vi "LeerBaseDatos_interno.vi"(8 "error in (no error)":errorcluster, 11 "Prueba01 in":refnum<class "Prueba01.lvclass">) -> (0 "error out":errorcluster, 3 "Prueba01 out":refnum<class "Prueba01.lvclass">)   [LabVIEW 2019, in "Prueba01.lvclass"]
uses:
  Prueba01.lvclass
  Controles/BD_P01.ctl
  Prueba01.lvclass/Prueba01.ctl
  Base de Datos/SQLiteConnector/SQLiteConnection.lvclass
  Base de Datos/Base de Datos.lvclass
panel:
  out "BD":T1
  in  "Tipo Equipo":enum16{"Sonometro", "Calibrador", "Dosimetro"}(ring)
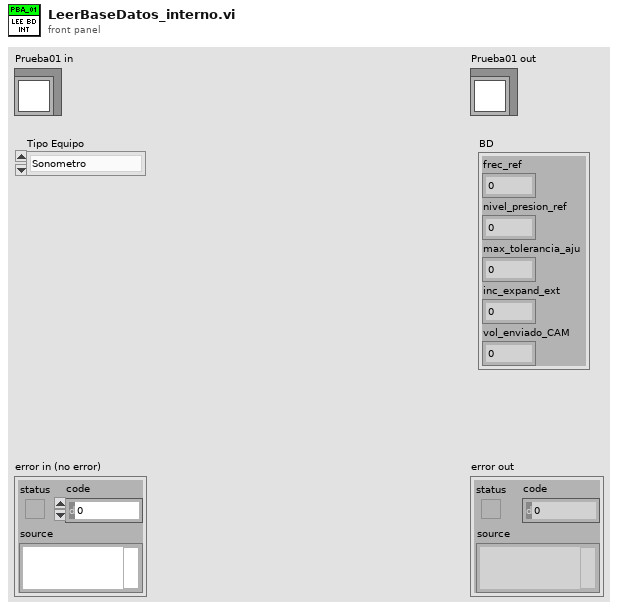
[diagram p1: front panel]
types:
  T1 = typedef "Prueba01.lvclass/BD_P01.ctl" = cluster{"frec_ref":dbl, "nivel_presion_ref":dbl, "max_tolerancia_aju":dbl, "inc_expand_ext":dbl, "vol_enviado_CAM":dbl}
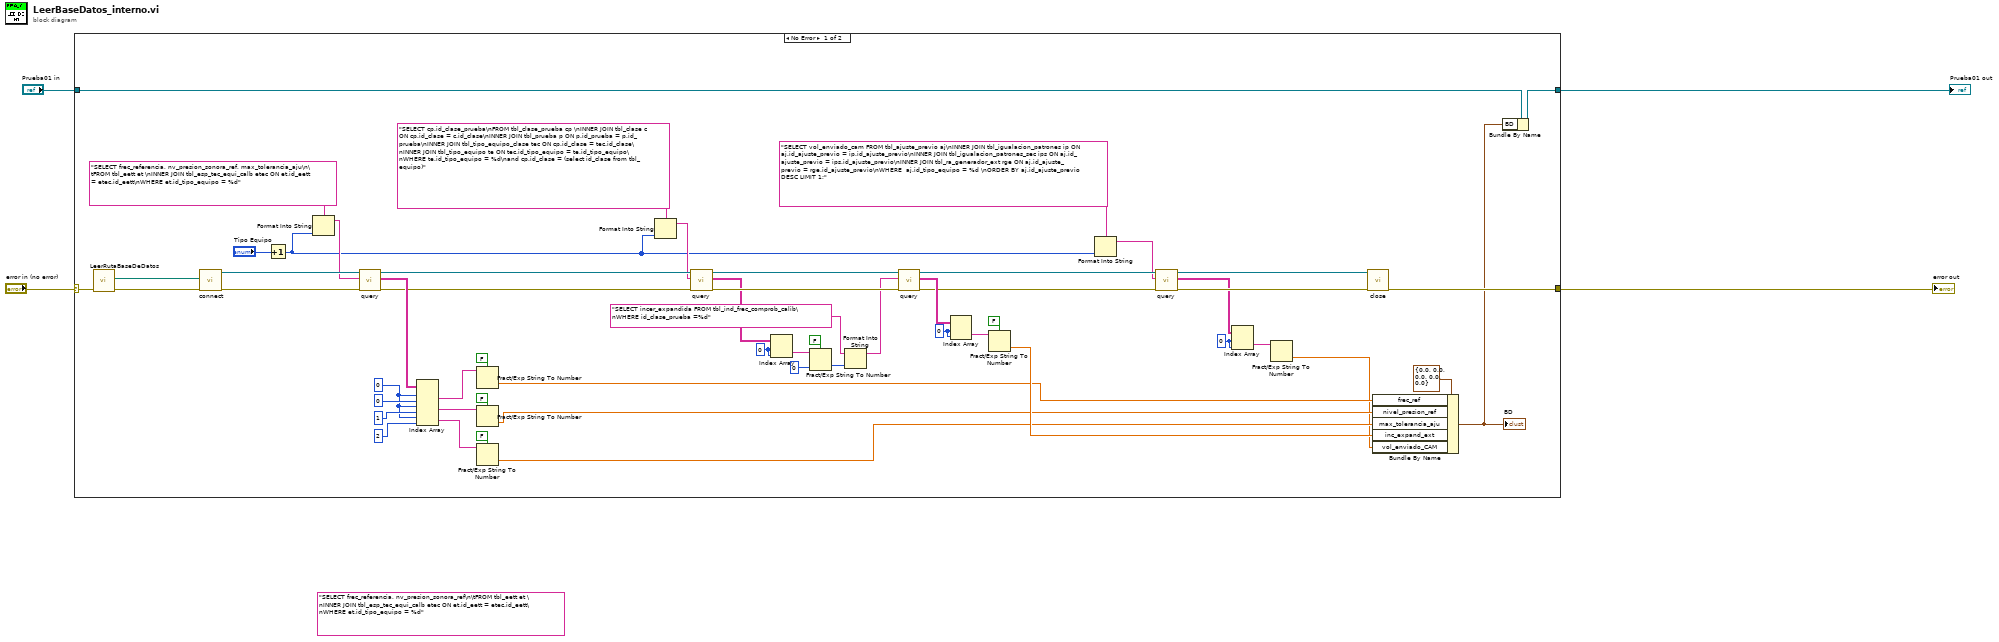
[diagram p0: block diagram]
diagram:
  (unwired) "SELECT frec_referencia, nv_presion_sonora_ref\n\tFROM tbl_eett et \nINNER JOIN tbl_esp_tec_equi_calb etec ON et.id_eett = etec.id_eett\nWHERE et.id_tipo_equipo = %d" ("format string")
  n1 = case shown="No Error" "error in (no error)" {
    selector: "error in (no error)" -> [w60 w63]
    tunnel: [w52 w63] -> w3
    tunnel: [w17 w62] -> w1
    tunnel: "Prueba01 in" -> [w61 w62]
    frame No Error {
      w8 = 0 ("index (row)")
      w24 = 0 ("index (row)")
      w35 = 0 ("index (row)")
      w44 = 0 ("index (row)")
      n2 = call "LeerRutaBaseDeDatos.vi"("error in (no error)"=w60) -> ("error out"=w54:errorcluster, "Database Path"=w53:path)  [unwired: 9 in]
      n3 = call "connect.vi"("error in (no error)"=w54, "Database Path"=w53) -> ("error out"=w56:errorcluster, "object out"=w57:refnum<class "SQLiteConnection.lvclass">)  [unwired: 8 in]
      n4 = Increment(x="Tipo Equipo") -> (x+1=w9:enum16{"Sonometro", "Calibrador", "Dosimetro"})
      n5 = Format Into String(format string="SELECT frec_referencia, nv_presion_sonora_ref, max_tolerancia_aju\n\tFROM tbl_eett et \nINNER JOIN tbl_esp_tec_equi_calb etec ON et.id_eett = etec.id_eett\nWHERE et.id_tipo_equipo = %d", w9) -> (resulting string=w55:string)  [unwired: 2 in, 1 out]
      n6 = call "query.vi"("error in (no error)"=w56, "SQL Statement"=w55, "object in"=w57) -> ("error out"=w40:errorcluster, "result"=w51:string[][], "object out"=w39:refnum<class "SQLiteConnection.lvclass">)  [unwired: 5 in, 1 out]
      n7 = Index Array(array=w51, index (row) #1=w44, index (col) #1=0 ("disabled index (col)"), index (row) #2=w44, index (col) #2=1 ("disabled index (col)"), index (row) #3=w44, index (col) #3=2 ("index (col)")) -> (element #1=w48:string, element #2=w47:string, element #3=w42:string)
      n8 = Fract/Exp String To Number(use system decimal point (T)=FALSE, string=w48) -> (number=w20:dbl)  [unwired: 2 in, 1 out]
      n9 = Fract/Exp String To Number(use system decimal point (T)=FALSE, string=w47) -> (number=w19:dbl)  [unwired: 2 in, 1 out]
      n10 = Fract/Exp String To Number(use system decimal point (T)=FALSE, string=w42) -> (number=w18:dbl)  [unwired: 2 in, 1 out]
      n11 = Format Into String(format string="SELECT cp.id_clase_prueba\nFROM tbl_clase_prueba cp \nINNER JOIN tbl_clase c ON cp.id_clase = c.id_clase\nINNER JOIN tbl_prueba p ON p.id_prueba = p.id_prueba\nINNER JOIN tbl_tipo_equipo_clase tec ON cp.id_clase = tec.id_clase\nINNER JOIN tbl_tipo_equipo te ON tec.id_tipo_equipo = te.id_tipo_equipo\nWHERE te.id_tipo_equipo = %d\nand cp.id_clase = (select id_clase from tbl_equipo)", w9) -> (resulting string=w37:string)  [unwired: 2 in, 1 out]
      n12 = call "query.vi"("error in (no error)"=w40, "SQL Statement"=w37, "object in"=w39) -> ("error out"=w36:errorcluster, "result"=w34:string[][], "object out"=w27:refnum<class "SQLiteConnection.lvclass">)  [unwired: 5 in, 1 out]
      n13 = Index Array(array=w34, index (row)=w35, index (col)=w35) -> (element=w32:string)
      n14 = Fract/Exp String To Number(use system decimal point (T)=FALSE, string=w32, default (0 dbl)=0 ("index (row)")) -> (number=w31:i32)  [unwired: 1 in, 1 out]
      n15 = Format Into String(format string="SELECT incer_expandida FROM tbl_ind_frec_comprob_calib\nWHERE id_clase_prueba =%d", w31) -> (resulting string=w28:string)  [unwired: 2 in, 1 out]
      n16 = call "query.vi"("error in (no error)"=w36, "SQL Statement"=w28, "object in"=w27) -> ("error out"=w14:errorcluster, "result"=w23:string[][], "object out"=w15:refnum<class "SQLiteConnection.lvclass">)  [unwired: 5 in, 1 out]
      n17 = Index Array(array=w23, index (row)=w24, index (col)=w24) -> (element=w26:string)
      n18 = Fract/Exp String To Number(use system decimal point (T)=FALSE, string=w26) -> (number=w21:dbl)  [unwired: 2 in, 1 out]
      n19 = Format Into String(format string="SELECT vol_enviado_cam FROM tbl_ajuste_previo aj\nINNER JOIN tbl_igualacion_patrones ip ON aj.id_ajuste_previo = ip.id_ajuste_previo\nINNER JOIN tbl_igualacion_patrones_sec ips ON aj.id_ajuste_previo = ips.id_ajuste_previo\nINNER JOIN tbl_ra_generador_ext rge ON aj.id_ajuste_previo = rge.id_ajuste_previo\nWHERE  aj.id_tipo_equipo = %d \nORDER BY aj.id_ajuste_previo DESC LIMIT 1;", w9) -> (resulting string=w10:string)  [unwired: 2 in, 1 out]
      n20 = call "query.vi"("error in (no error)"=w14, "SQL Statement"=w10, "object in"=w15) -> ("error out"=w12:errorcluster, "result"=w6:string[][], "object out"=w13:refnum<class "SQLiteConnection.lvclass">)  [unwired: 5 in, 1 out]
      n21 = Index Array(array=w6, index (row)=w8, index (col)=w8) -> (element=w7:string)
      n22 = Fract/Exp String To Number(string=w7) -> (number=w5:dbl)  [unwired: 3 in, 1 out]
      n23 = call-dynamic "close.vi"("error in (no error)"=w12, "object in"=w13) -> ("error out"=w52:errorcluster)  [unwired: 8 in, 1 out]
      n24 = Bundle By Name(cluster=T1 {"frec_ref"=0.0, "nivel_presion_ref"=0.0, "max_tolerancia_aju"=0.0, "inc_expand_ext"=0.0, "vol_enviado_CAM"=0.0}, "frec_ref"=w20, "nivel_presion_ref"=w19, "max_tolerancia_aju"=w18, "inc_expand_ext"=w21, "vol_enviado_CAM"=w5) -> (w16:T1)
      "BD" <- w16
      n25 = Bundle By Name(cluster=w61, "BD"=w16) -> (w17:refnum<class "Prueba01.lvclass">)
    }
    frame Error {
    }
  }
  "error out" <- w3
  "Prueba01 out" <- w1
